vi "Joystick to Arcade.vi"(7 "Negate Right input (true)":bool=TRUE, 10 "Forward":dbl format="%#_13g", 11 "Right":dbl format="%#_13g") -> (2 "Right Wheel":dbl format="%#_13g", 3 "Left Wheel":dbl format="%#_13g")   [LabVIEW 2019]
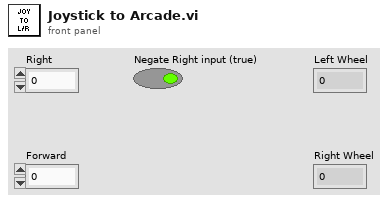
[diagram p1: front panel]
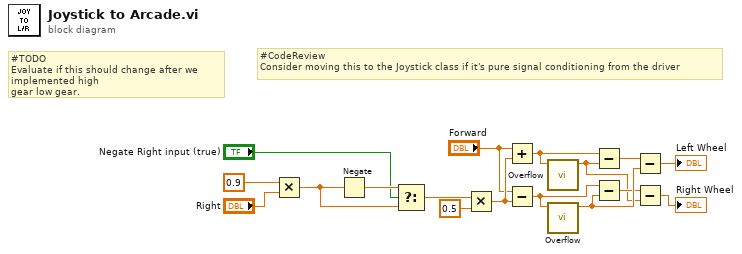
[diagram p0: block diagram]
diagram:
  # "#CodeReview\nConsider moving this to the Joystick class if it's pure signal conditioning from the driver"
  # "#TODO\nEvaluate if this should change after we implemented high\ngear low gear."
  n1 = Multiply(x=0.9, y="Right") -> (x*y=w2:dbl)
  n2 = Negate(x=w2) -> (-x=w6:dbl)
  n3 = Select(t=w6, s="Negate Right input (true)", f=w2) -> (s? t:f=w5:dbl)
  n4 = Multiply(x=w5, y=0.5) -> (x*y=w16:dbl)
  n5 = Add(x="Forward", y=w16) -> (x+y=w14:dbl)
  n6 = Subtract(x="Forward", y=w16) -> (x-y=w11:dbl)
  n7 = call "Overflow.vi"("Value"=w14) -> ("Overflow"=w8:dbl)  [unwired: 10 in]
  n8 = call "Overflow.vi"("Value"=w11) -> ("Overflow"=w10:dbl)  [unwired: 10 in]
  n9 = Subtract(x=w14, y=w8) -> (x-y=w13:dbl)
  n10 = Subtract(x=w11, y=w10) -> (x-y=w9:dbl)
  n11 = Subtract(x=w13, y=w10) -> (x-y=→"Left Wheel":dbl)
  n12 = Subtract(x=w9, y=w8) -> (x-y=→"Right Wheel":dbl)
